vi "calibAnnotate.vi"(5 "Image height":u32, 7 "Image width":u32, 9 "Side border":dbl, 10 "Bottom border":dbl, 11 "Image":T1) -> (3 "Image Out":T1)   [LabVIEW 2020]
uses:
  <vilib>/vision/Image Controls.llb/IMAQ Image.ctl
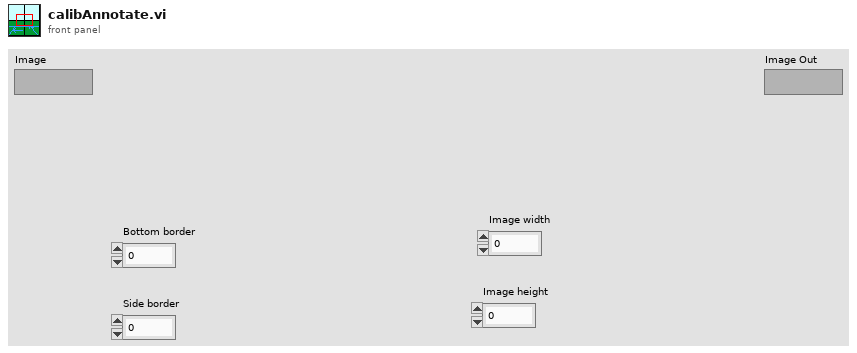
[diagram p1: front panel]
types:
  T1 = typedef "IMAQ Image.ctl" = refnum<image>
  T2 = cluster{"Desired Font (Application)":enum16{"User-specified Font", "Application Font", "System Font", "Dialog Font"}, "[User-specified Font]":cluster{"Font Name":string, "Size":i16, "Strikeout?":bool, "Italic?":bool, "Underline?":bool, "Outline?":bool, "Shadow?":bool, "Bold?":bool, "Rotation Angle":dbl}, "Horizontal Alignment":i16, "Vertical Alignment":i16}
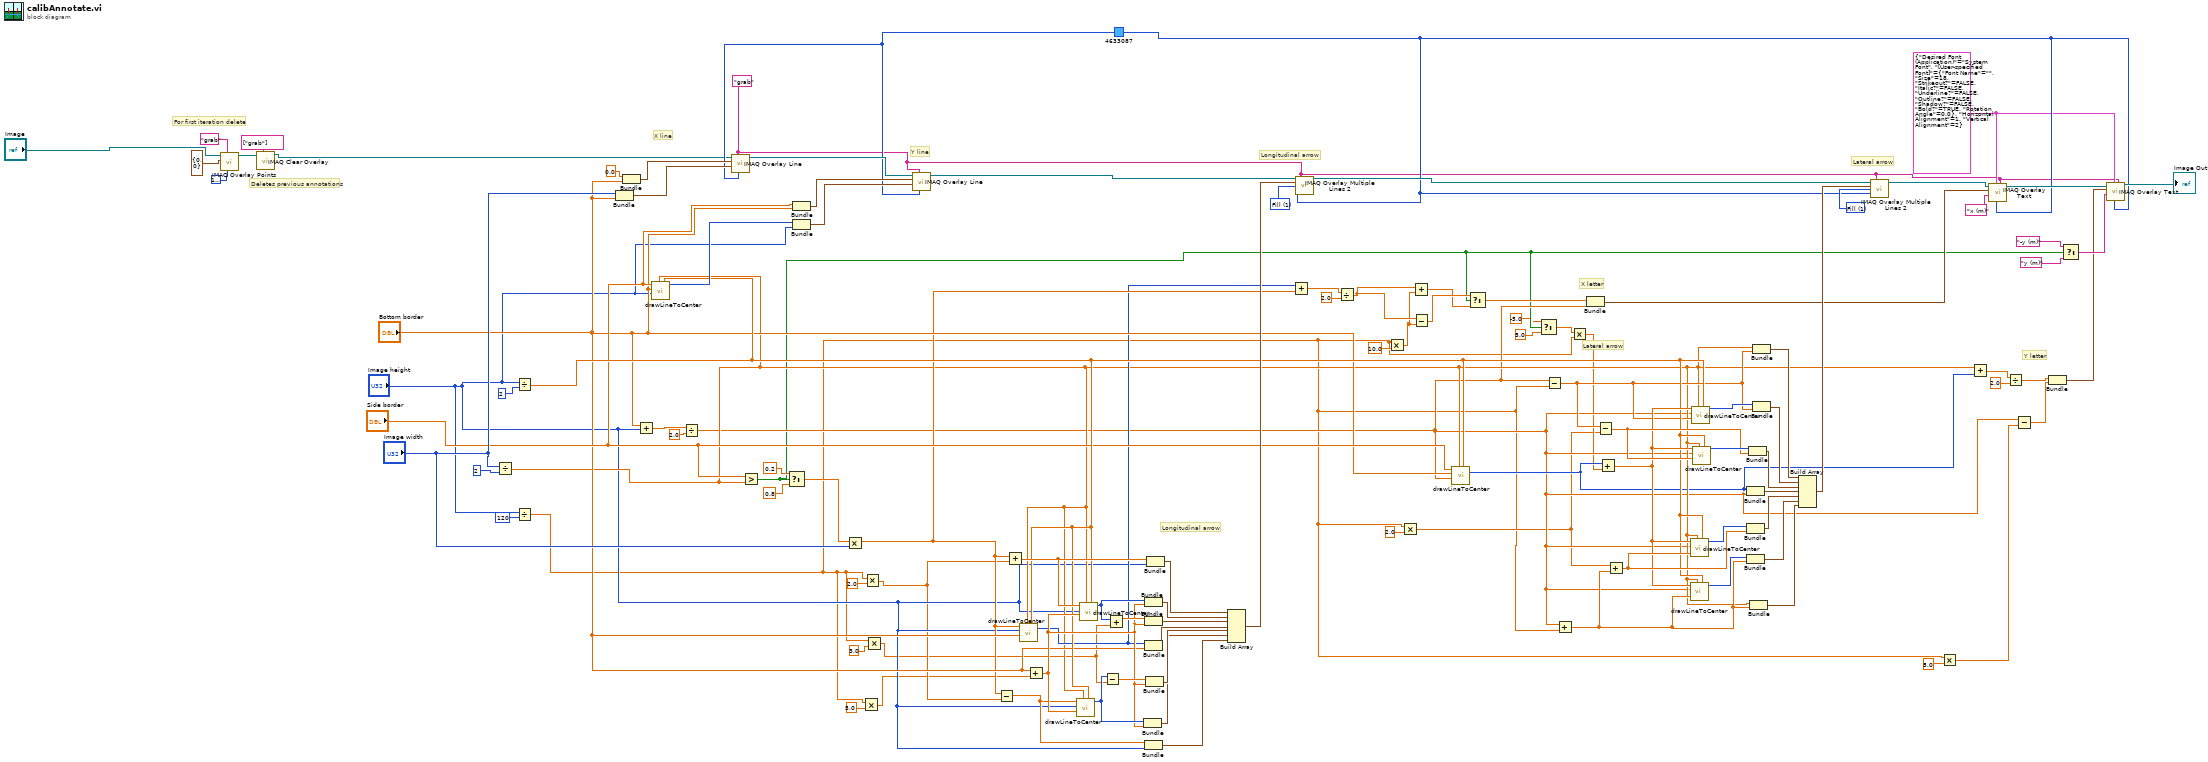
[diagram p0: block diagram]
diagram:
  w8 = "grab" ("Group")
  w29 = T2 {"Desired Font (Application)"=enum."System Font", "[User-specified Font]"={"Font Name"="", "Size"=18, "Strikeout?"=FALSE, "Italic?"=FALSE, "Underline?"=FALSE, "Outline?"=FALSE, "Shadow?"=FALSE, "Bold?"=TRUE, "Rotation Angle"=0.0}, "Horizontal Alignment"=1, "Vertical Alignment"=2} ("Font, Size & Style")
  w68 = u32 1 items=["Frame", "Fill"] ("Drawing Mode (Frame)")
  w102 = u32 1 items=["Frame", "Fill"] ("Drawing Mode (Frame)")
  w47 = u32 4633087 ("Color")
  # "For first iteration delete"
  # "Deletes previous annotations"
  # "Y letter"
  # "X letter"
  # "Lateral arrow"
  # "Longitudinal arrow"
  # "X line"
  # "Y line"
  # "Lateral arrow"
  # "Longitudinal arrow"
  n1 = call "IMAQ Overlay Points"("Color"=u32 16777216, "Group"="grab", "Point"=cluster{"X":i32, "Y":i32} {"X"=0, "Y"=0}, "Image"="Image") -> ("Image Out"=w3:T1)  [unwired: 6 in, 1 out]
  n2 = call "IMAQ Clear Overlay"("Groups"=string[] ["grab"], "Image"=w3) -> ("Image Out"=w1:T1)  [unwired: 8 in, 1 out]
  n3 = Divide(x="Image width", y=u32 2) -> (x/y=w35:dbl)
  n4 = Divide(x="Image height", y=u32 2) -> (x/y=w59:dbl)
  n5 = Divide(x="Image height", y=u32 120) -> (x/y=w9:dbl)
  n6 = Bundle("Image width"="Image width", "Bottom border"="Bottom border") -> (w105:cluster{"Image width":u32, "Bottom border":dbl})  [unwired: 1 in]
  n7 = Bundle(0.0, "Bottom border"="Bottom border") -> (w106:cluster{dbl, "Bottom border":dbl})  [unwired: 1 in]
  n8 = Add(x="Bottom border", y="Image height") -> (x+y=w85:dbl)
  n9 = call "drawLineToCenter.vi"("ycenter"=w59, "xcenter"=w35, "yend"="Image height", "ystart"="Bottom border", "xstart"="Side border") -> ("xend"=w65:i32)  [unwired: 6 in]
  n10 = Divide(x=w85, y=2.0) -> (x/y=w30:dbl)
  n11 = call "IMAQ Overlay Line"("Color"=w47, "Group"=w8, "End Point"=w105, "Start Point"=w106, "Image"=w1) -> ("Image Out"=w108:T1)  [unwired: 5 in, 1 out]
  n12 = Greater?(x="Side border", y=w35) -> (0:w28:bool)
  n13 = Select(t=0.2, s=w28, f=0.8) -> (s? t:f=w61:dbl)
  n14 = Bundle("Side border"="Side border", "Bottom border"="Bottom border") -> (w66:cluster{"Side border":dbl, "Bottom border":dbl})  [unwired: 1 in]
  n15 = Bundle("xend"=w65, "Image height"="Image height") -> (w67:cluster{"xend":i32, "Image height":u32})  [unwired: 1 in]
  n16 = Multiply(x=w61, y="Image width") -> (x*y=w44:dbl)
  n17 = Multiply(x=w9, y=5.0) -> (x*y=w18:dbl)
  n18 = Multiply(x=w9, y=2.0) -> (x*y=w22:dbl)
  n19 = Multiply(x=w9, y=3.0) -> (x*y=w19:dbl)
  n20 = call "IMAQ Overlay Line"("Color"=w47, "Group"=w8, "End Point"=w67, "Start Point"=w66, "Image"=w108) -> ("Image Out"=w100:T1)  [unwired: 5 in, 1 out]
  n21 = Subtract(x=w44, y=w22) -> (x-y=w62:dbl)
  n22 = Add(x=w44, y=w22) -> (x+y=w88:dbl)
  n23 = call "drawLineToCenter.vi"("ycenter"=w59, "xcenter"=w35, "yend"="Bottom border", "ystart"="Image height", "xstart"=w44) -> ("xend"=w43:i32)  [unwired: 6 in]
  n24 = Add(x="Bottom border", y=w18) -> (x+y=w87:dbl)
  n25 = call "drawLineToCenter.vi"("ycenter"=w59, "xcenter"=w35, "yend"=w87, "ystart"="Image height", "xstart"=w62) -> ("xend"=w93:i32)  [unwired: 6 in]
  n26 = call "drawLineToCenter.vi"("ycenter"=w59, "xcenter"=w35, "yend"=w87, "ystart"="Image height", "xstart"=w88) -> ("xend"=w99:i32)  [unwired: 6 in]
  n27 = Subtract(x=w93, y=w19) -> (x-y=w92:dbl)
  n28 = Add(x=w99, y=w19) -> (x+y=w98:dbl)
  n29 = Bundle("xend"=w93, w87) -> (w90:cluster{"xend":i32, dbl})  [unwired: 1 in]
  n30 = Bundle(w62, "Image height"="Image height") -> (w89:cluster{dbl, "Image height":u32})  [unwired: 1 in]
  n31 = Bundle("xend"=w99, w87) -> (w96:cluster{"xend":i32, dbl})  [unwired: 1 in]
  n32 = Bundle(w98, w87) -> (w95:cluster{dbl, dbl})  [unwired: 1 in]
  n33 = Bundle("xend"=w43, "Bottom border"="Bottom border") -> (w94:cluster{"xend":i32, "Bottom border":dbl})  [unwired: 1 in]
  n34 = Bundle(w92, w87) -> (w91:cluster{dbl, dbl})  [unwired: 1 in]
  n35 = Bundle(w88, "Image height"="Image height") -> (w97:cluster{dbl, "Image height":u32})  [unwired: 1 in]
  n36 = Build Array(w97, w96, w95, w94, w91, w90, w89) -> (w101:cluster{"xend":dbl, "Bottom border":dbl}[])
  n37 = Add(x=w43, y=w44) -> (x+y=w45:dbl)
  n38 = call "IMAQ Overlay Multiple Lines 2"("Image"=w100, "Group"=w8, "Line End Points"=w101, "Drawing Mode (Frame)"=w102, "Color"=w47) -> ("Image Out"=w86:T1)  [unwired: 9 in, 1 out]
  n39 = Divide(x=w45, y=2.0) -> (x/y=w42:dbl)
  n40 = Multiply(x=w9, y=10.0) -> (x*y=w15:dbl)
  n41 = Multiply(x=w9, y=2.0) -> (x*y=w12:dbl)
  n42 = Add(x=w42, y=w15) -> (x+y=w40:dbl)
  n43 = Subtract(x=w42, y=w15) -> (x-y=w41:dbl)
  n44 = call "drawLineToCenter.vi"("ycenter"=w59, "xcenter"=w35, "yend"=w30, "ystart"="Bottom border", "xstart"="Side border") -> ("xend"=w34:i32)  [unwired: 6 in]
  n45 = Select(t=w41, s=w28, f=w40) -> (s? t:f=w39:dbl)
  n46 = Select(t=-5.0, s=w28, f=5.0) -> (s? t:f=w14:dbl)
  n47 = Subtract(x=w30, y=w9) -> (x-y=w56:dbl)
  n48 = Add(x=w30, y=w9) -> (x+y=w55:dbl)
  n49 = Multiply(x=w14, y=w9) -> (x*y=w13:dbl)
  n50 = Bundle(w39, w30) -> (w38:cluster{dbl, dbl})  [unwired: 1 in]
  n51 = Subtract(x=w56, y=w12) -> (x-y=w81:dbl)
  n52 = Add(x=w34, y=w13) -> (x+y=w72:dbl)
  n53 = Add(x=w12, y=w55) -> (x+y=w75:dbl)
  n54 = call "drawLineToCenter.vi"("ycenter"=w59, "xcenter"=w35, "yend"=w75, "ystart"=w30, "xstart"=w72) -> ("xend"=w76:i32)  [unwired: 6 in]
  n55 = call "drawLineToCenter.vi"("ycenter"=w59, "xcenter"=w35, "yend"=w55, "ystart"=w30, "xstart"=w72) -> ("xend"=w73:i32)  [unwired: 6 in]
  n56 = call "drawLineToCenter.vi"("ycenter"=w59, "xcenter"=w35, "yend"=w56, "ystart"=w30, "xstart"=w72) -> ("xend"=w83:i32)  [unwired: 6 in]
  n57 = call "drawLineToCenter.vi"("ycenter"=w59, "xcenter"=w35, "yend"=w81, "ystart"=w30, "xstart"=w72) -> ("xend"=w82:i32)  [unwired: 6 in]
  n58 = Bundle("xend"=w34, w30) -> (w77:cluster{"xend":i32, dbl})  [unwired: 1 in]
  n59 = Bundle("xend"=w76, w75) -> (w74:cluster{"xend":i32, dbl})  [unwired: 1 in]
  n60 = Bundle("xend"=w73, w55) -> (w70:cluster{"xend":i32, dbl})  [unwired: 1 in]
  n61 = Bundle("xend"=w82, w81) -> (w78:cluster{"xend":i32, dbl})  [unwired: 1 in]
  n62 = Bundle(w35, w55) -> (w71:cluster{dbl, dbl})  [unwired: 1 in]
  n63 = Bundle(w35, w56) -> (w80:cluster{dbl, dbl})  [unwired: 1 in]
  n64 = Bundle("xend"=w83, w56) -> (w79:cluster{"xend":i32, dbl})  [unwired: 1 in]
  n65 = Build Array(w80, w79, w78, w77, w74, w70, w71) -> (w69:cluster{"xend":dbl, dbl}[])
  n66 = call "IMAQ Overlay Multiple Lines 2"("Image"=w86, "Group"=w8, "Line End Points"=w69, "Drawing Mode (Frame)"=w68, "Color"=w47) -> ("Image Out"=w53:T1)  [unwired: 9 in, 1 out]
  n67 = Multiply(x=w9, y=5.0 ("x")) -> (x*y=w11:dbl)
  n68 = Add(x=w35, y=w34) -> (x+y=w36:dbl)
  n69 = call "IMAQ Overlay Text"("Group"=w8, "Text Color (black)"=w47, "Font, Size & Style"=w29, "String"="x (m)", "Origin"=w38, "Image"=w53) -> ("Image Out"=w52:T1)  [unwired: 4 in, 1 out]
  n70 = Divide(x=w36, y=2.0) -> (x/y=w33:dbl)
  n71 = Subtract(x=w30, y=w11) -> (x-y=w32:dbl)
  n72 = Bundle(w33, w32) -> (w31:cluster{dbl, dbl})  [unwired: 1 in]
  n73 = Select(t="-y (m)", s=w28, f="y (m)") -> (s? t:f=w50:string)
  n74 = call "IMAQ Overlay Text"("Group"=w8, "Text Color (black)"=w47, "Font, Size & Style"=w29, "String"=w50, "Origin"=w31, "Image"=w52) -> ("Image Out"=→"Image Out":T1)  [unwired: 4 in, 1 out]
